vi "HTML Formatted String.vi"(7 "Str Refnum":refnum<vi>, 10 "Message":string) -> ()   [LabVIEW 2020, in "Multiple Errors.lvclass"]
uses:
  Multiple Errors.lvclass
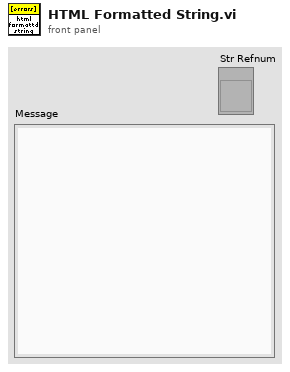
[diagram p1: front panel]
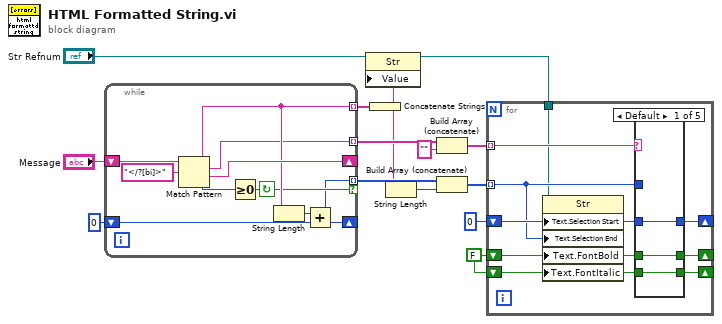
[diagram p0: block diagram]
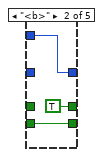
[diagram p2: hidden frame]
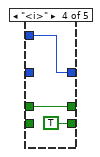
[diagram p4: hidden frame]
diagram:
  w8 = FALSE ("Text.Font:Bold")
  n1 = while {
    shift-right: [w22] -> _
    shift-left: "Message" -> [w23]
    tunnel: [w21] -> w12 mode=indexing
    shift-right: [w16] -> _
    shift-left: 0 -> [w18]
    tunnel: [w16] -> w9 mode=indexing if=w17
    tunnel: [w15] -> w11 mode=indexing
    stop <- w17 continue-if-true
    n2 = Match Pattern(string=w23, regular expression="</?[bi]>") -> (before substring=w21:string, match substring=w15:string, after substring=w22:string, offset past match=w19:i32)  [unwired: 1 in]
    n3 = Greater Or Equal To 0?(x=w19) -> (x >= 0?=w17:bool)
    n4 = String Length(string=w21) -> (length=w20:i32)
    n5 = Add(x=w20, y=w18) -> (x+y=w16:i32)
  }
  n6 = Concatenate Strings(w12) -> (w1:string)
  n7 = property class="Str"(reference="Str Refnum", "Value"=w1) -> (reference out=w6:refnum<vi>)  [unwired: 1 in, 1 out]
  n8 = String Length(string=w1) -> (length=w2:i32)
  n9 = Build Array (concatenate)(w11, "" ("element")) -> (w5:string[])
  n10 = Build Array (concatenate)(w9, w2) -> (w4:i32[])
  n11 = for {
    tunnel: w5 -> [w33] mode=indexing
    shift-right: [w31] -> _
    shift-left: 0 -> [w29]
    shift-right: [w32] -> _
    shift-left: w8 -> [w27]
    tunnel: w4 -> [w28] mode=indexing
    shift-right: [w30] -> _
    shift-left: w8 -> [w26]
    tunnel: w6 -> [w25]
    n12 = property on="Property Node" class="Str"(reference=w25, "Text.Selection Start"=w29, "Text.Selection End"=w28, "Text.FontBold"=w27, "Text.FontItalic"=w26) -> ()  [unwired: 1 in, 2 out]
    n13 = case shown="Default" w33 {
      tunnel: w28 -> [_ w39 w41 w44 w46]
      tunnel: w29 -> [w36 _ _ _ _]
      tunnel: w27 -> [w35 _ _ w43 w45]
      tunnel: [w35 TRUE ("Text.Font:Bold") _ w43 w45] -> w32
      tunnel: [w36 w39 w41 w44 w46] -> w31
      tunnel: w26 -> [w34 w38 w40 _ _]
      tunnel: [w34 w38 w40 TRUE ("Text.Font:Bold") _] -> w30
      frame Default {
      }
      frame "<b>" {
      }
      frame "</b>" {
      }
      frame "<i>" {
      }
      frame "</i>" {
      }
    }
  }
